vi "MOTOR Action-Status Position.vi"(8 "error in (no error)":errorcluster, 10 "Message Data":variant, 11 "Data Cluster in":T1={"Tango HW"={"VISA resource"="", "Baud Rate (115200)"=2, "lAnInterfaceType"=0, "bAShowProt"=15}, "Writer Queue"=refnum, "Status"=FALSE, "Abs Position"=[], "Axis Velocity"={"dX"=0.0, "dY"=0.0, "dZ"=0.0, "dA"=0.0}, "acceleration "=0.0, "Z direction"=enum."Up", "Position Mode"="", "plLSID"=0}) -> (0 "error out":errorcluster, 3 "Data Cluster out":T1={"Tango HW"={"VISA resource"="", "Baud Rate (115200)"=2, "lAnInterfaceType"=0, "bAShowProt"=15}, "Writer Queue"=refnum, "Status"=FALSE, "Abs Position"=[], "Axis Velocity"={"dX"=0.0, "dY"=0.0, "dZ"=0.0, "dA"=0.0}, "acceleration "=0.0, "Z direction"=enum."Up", "Position Mode"="", "plLSID"=0})   [LabVIEW 2020, in "MOTOR.lvlib"]
uses:
  MOTOR.lvlib
  PS Hardware Configuration.ctl
  support/Message Queue/Message Cluster.ctl
  support/HW Message Cluster.ctl
  support/PCT FGV CMD.ctl
  support/Message Queue/Enqueue Message (Single).vi
  support/Message Queue/Message Queue.lvlib
  <instrlib>/Tango_DLL/Tango_DLL.lvlib
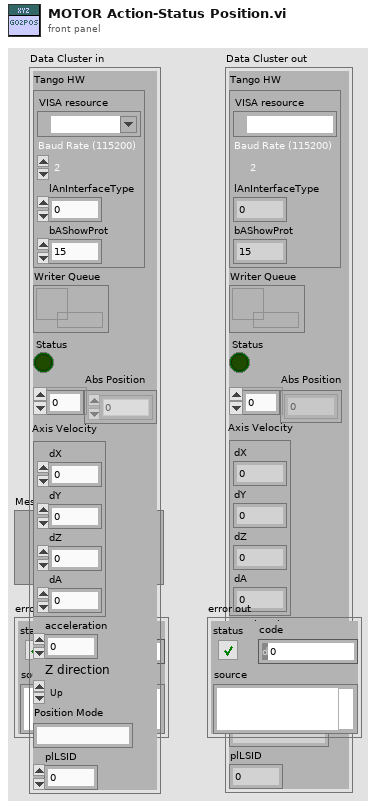
[diagram p1: front panel]
types:
  T1 = typedef "MOTOR.lvlib/PS Hardware Configuration.ctl" = cluster{"Tango HW":cluster{"VISA resource":refnum<visa-resource-name>, "Baud Rate (115200)":i32, "lAnInterfaceType":i32, "bAShowProt":i32}, "Writer Queue":refnum<queue>, "Status":bool, "Abs Position":i32[], "Axis Velocity":cluster{"dX":dbl, "dY":dbl, "dZ":dbl, "dA":dbl}, "acceleration ":dbl, "Z direction":enum16{"Up", "Down"}, "Position Mode":string, "plLSID":i32}
  T2 = typedef "PCT FGV CMD.ctl" = enum16{"INIT", "GET", "SET"}
  T3 = typedef "Message Queue.lvlib/HW Message Cluster.ctl" = cluster{"Writer Queue":refnum<queue>, "Writer Data":T4}
  T4 = typedef "Message Queue.lvlib/Message Cluster.ctl" = cluster{"Message":string, "Message Data":variant}
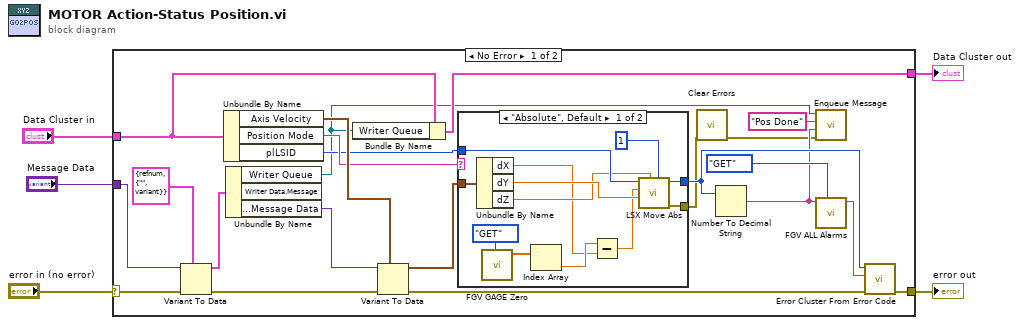
[diagram p0: block diagram]
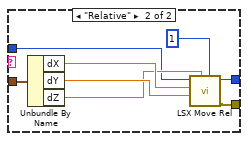
[diagram p2: hidden frame]
diagram:
  n1 = case shown="No Error" "error in (no error)" {
    selector: "error in (no error)" -> [w20 w48]
    tunnel: "Message Data" -> [w19 _]
    tunnel: [w18 w49] -> w4
    tunnel: "Data Cluster in" -> [w21 w49]
    tunnel: [w15 w48] -> w2
    frame No Error {
      n2 = Variant To Data(error in=w20, type=T3 {"Writer Queue"=refnum, "Writer Data"={"Message"="", "Message Data"=variant}}, Variant=w19) -> (data=w22:T3, error out=w24:errorcluster)
      n3 = Unbundle By Name(w21) -> ("Axis Velocity"=w26:cluster{"dX":dbl, "dY":dbl, "dZ":dbl, "dA":dbl}, "Position Mode"=w13:string, "plLSID"=w12:i32)
      n4 = Unbundle By Name(w22) -> ("Writer Queue"=w9:refnum<queue>, "Writer Data.Message Data"=w23:variant)  [unwired: 1 out]
      n5 = Bundle By Name(cluster=w21, "Writer Queue"=w9) -> (w18:T1)
      n6 = Variant To Data(error in=w24, type=w26, Variant=w23) -> (data=w17:cluster{"dX":dbl, "dY":dbl, "dZ":dbl, "dA":dbl}, error out=w27:errorcluster)
      n7 = case shown="\"Absolute\", Default" w13 {
        tunnel: w17 -> [w39 w47]
        tunnel: w12 -> [w38 w43]
        tunnel: [w34 w41] -> w11
        tunnel: [w33 w40] -> w7
        frame "Absolute", Default {
          n8 = Unbundle By Name(w39) -> ("dX"=w29:dbl, "dY"=w37:dbl, "dZ"=w36:dbl)
          n9 = call "FGV GAGE Zero.vi"("CMD"=PCT_FGV_CMD."GET") -> ("output"=w31:dbl[])  [unwired: 9 in, 1 out]
          n10 = Index Array(array=w31) -> (element=w30:dbl)  [unwired: 1 in]
          n11 = Subtract(x=w30, y=w29) -> (x-y=w28:dbl)
          n12 = call <instrlib>:"LSX Move Abs.vi"("bWait"=1, "dZ"=w36, "dY"=w37, "dX"=w28, "lLSID"=w38) -> ("error out"=w33:errorcluster, "function return"=w34:i32)  [unwired: 5 in]
        }
        frame "Relative" {
          n13 = Unbundle By Name(w47) -> ("dX"=w46:dbl, "dY"=w45:dbl, "dZ"=w44:dbl)
          n14 = call <instrlib>:"LSX Move Rel.vi"("bWait"=1, "dZ"=w44, "dY"=w45, "dX"=w46, "lLSID"=w43) -> ("error out"=w40:errorcluster, "function return"=w41:i32)  [unwired: 5 in]
        }
      }
      n15 = call <vilib>:"Clear Errors.vi"("error in (no error)"=w7) -> ("error out"=w6:errorcluster)  [unwired: 5 in, 1 out]
      n16 = Number To Decimal String(number=w11) -> (decimal integer string=w8:string)  [unwired: 1 in]
      n17 = call-poly "Enqueue Message.vi"("error in (no error)"=w6, "Message Data"=w8, "Message"="Pos Done", "Message Queue"=w9) -> ()  [unwired: 6 in, 2 out]
      n18 = call "FGV ALL Alarms.vi"("CMD"=PCT_FGV_CMD."GET", "name"=w8) -> ("Alarm MSG out"=w14:string)  [unwired: 8 in, 1 out]
      n19 = call <vilib>:"Error Cluster From Error Code.vi"("error in (no error)"=w27, "error message (\"\")"=w14, "error code (0)"=w11) -> ("error out"=w15:errorcluster)  [unwired: 6 in]
    }
    frame Error {
    }
  }
  "Data Cluster out" <- w4
  "error out" <- w2
